vi "Start Calibrate.vi"(0 "CART TCP Connection In":refnum<k5>, 5 "Send Cal Command?":bool=TRUE, 7 "Calibrate Config":T1={"Frequency, MHz"=2412, "TX Gain"=0, "Data Rate"="1,0,0", "Packet Length"=4, "Packet Count"=4}, 11 "error in (no error)":errorcluster) -> (4 "CART TCP Connection Out":refnum<k5>, 6 "Messages Logged":string[](array[string]), 8 "More Pwr Reporting?":bool, 14 "Command Sent":string, 15 "error out":errorcluster)   [LabVIEW 2011]
uses:
  WLAN/UUT/QCA/Controls/QCA NART Response Type.ctl
  WLAN/UUT/QCA/NART Constants.vi
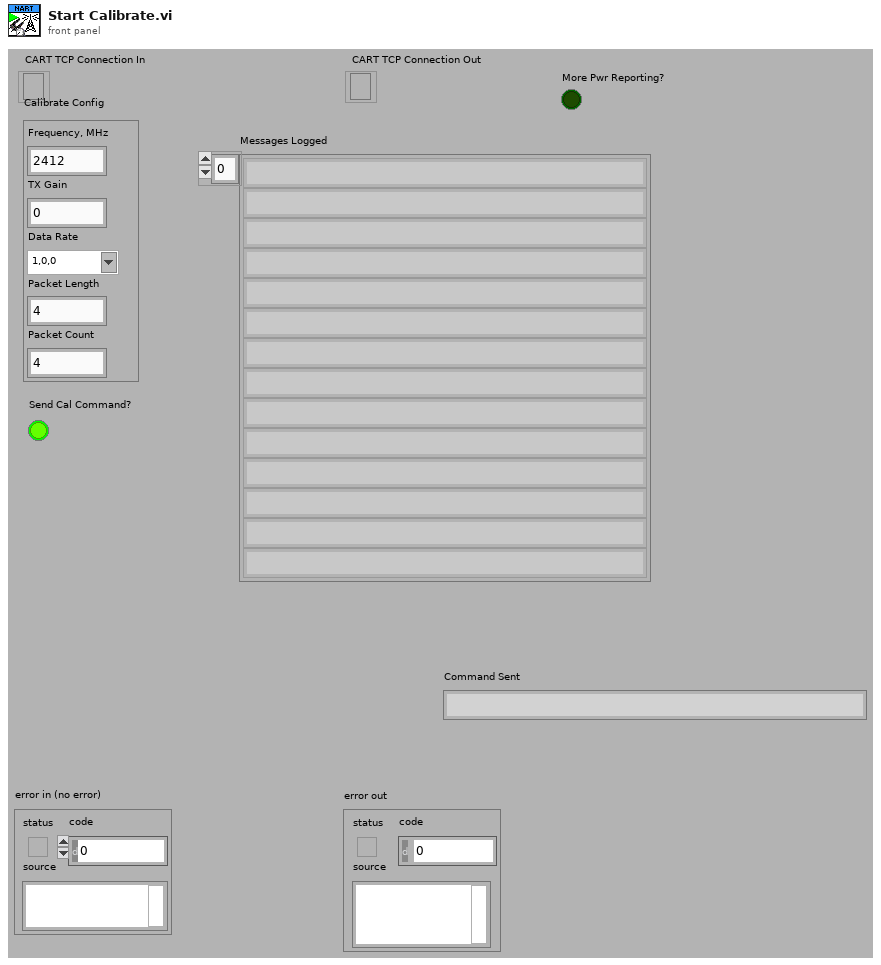
[diagram p1: front panel]
types:
  T1 = cluster{"Frequency, MHz":u32, "TX Gain":u32, "Data Rate":string, "Packet Length":u32, "Packet Count":i32}
  T2 = typedef "QCA NART Response Type.ctl" = enum16{"DEBUG", "CONTROL", "INFO", "WARNING", "ERROR", "NONE"}
  T3 = enum16{"none", "combined", "isolated", "iterate-combined ", "iterate-isolated"}
  T4 = cluster{"Name":string, "Type":enum16{"decimal", "string", "float", "hex"}}[]
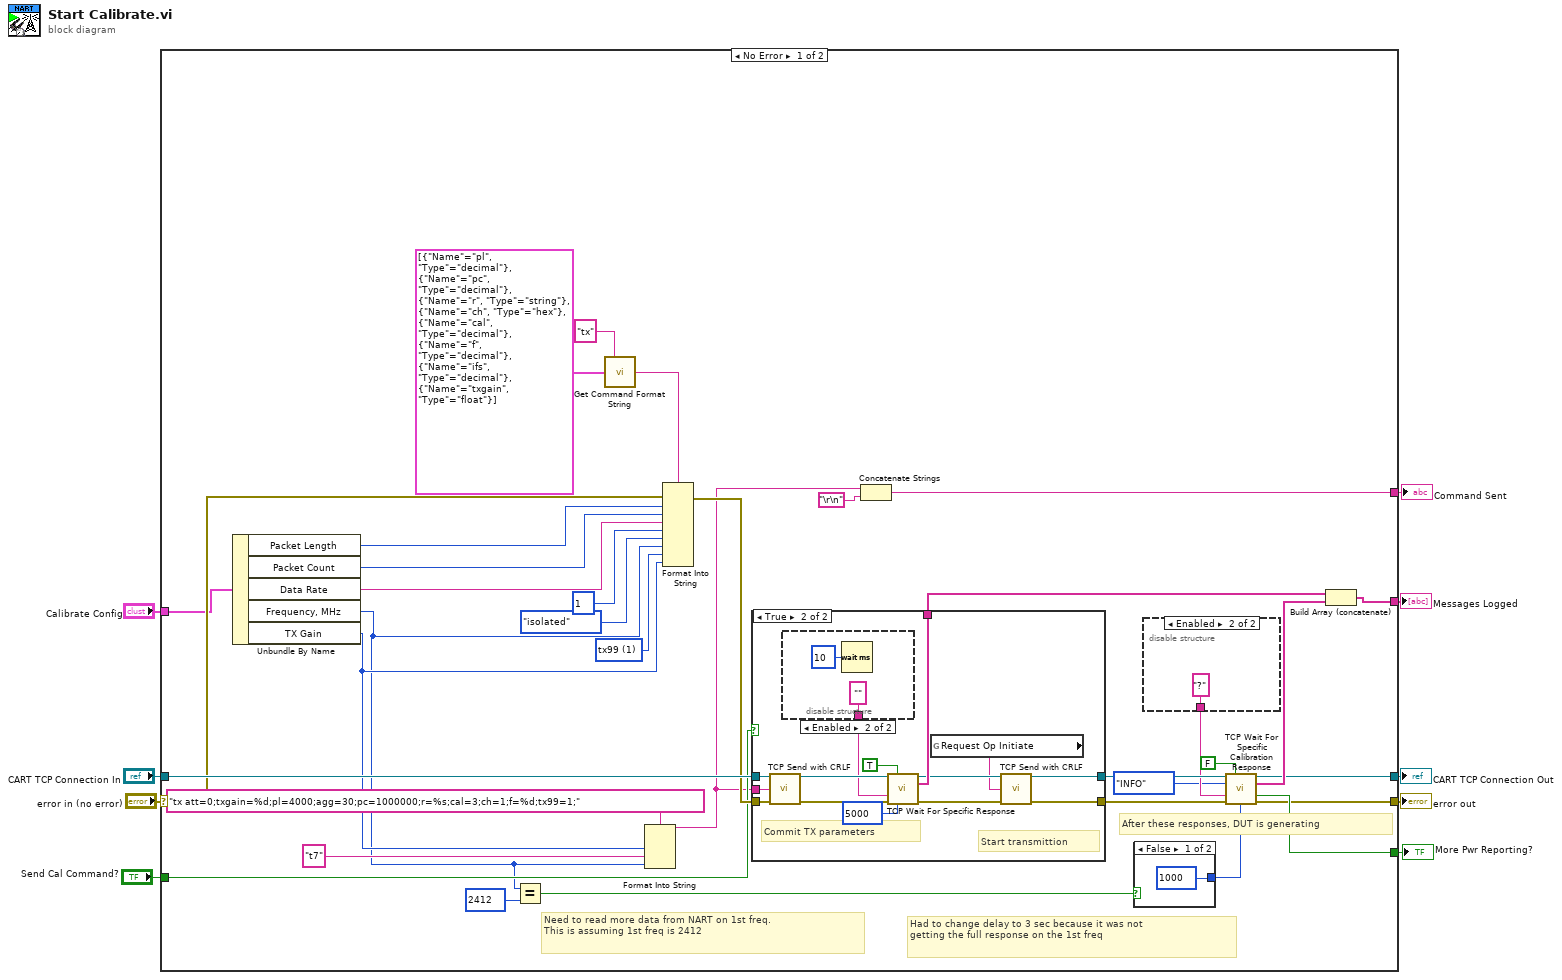
[diagram p0: block diagram]
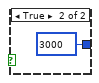
[diagram p2: hidden frame]
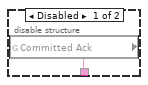
[diagram p4: hidden frame]
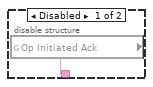
[diagram p5: hidden frame]
diagram:
  n1 = case shown="No Error" "error in (no error)" {
    selector: "error in (no error)" -> [w43 w69]
    tunnel: [w15 w69] -> w8
    tunnel: "CART TCP Connection In" -> [w44 w68]
    tunnel: [w16 w68] -> w6
    tunnel: "Calibrate Config" -> [w41 _]
    tunnel: [w37 _] -> w4
    tunnel: [w30 _] -> w3
    tunnel: [w18 _] -> w2
    tunnel: "Send Cal Command?" -> [w14 _]
    frame No Error {
      w28 = i16 1 items=["Regular"=-1, "tx100"=0, "tx99"=1] ("Inter Frame Spacing")
      # "Need to read more data from NART on 1st freq.\nThis is assuming 1st freq is 2412"
      # "Had to change delay to 3 sec because it was not \ngetting the full response on the 1st freq"
      # "After these responses, DUT is generating"
      n2 = Unbundle By Name(w41) -> ("Packet Length"=w40:u32, "Packet Count"=w34:i32, "Data Rate"=w21:string, "Frequency, MHz"=w12:u32, "TX Gain"=w22:u32)
      n3 = Equal?(x=w12, y=2412) -> (x = y?=w11:bool)
      n4 = call "Get Command Format String.vi"("Command"="tx", "Parameters"=T4 [{"Name"="pl", "Type"=enum."decimal"}, {"Name"="pc", "Type"=enum."decimal"}, {"Name"="r", "Type"=enum."string"}, {"Name"="ch", "Type"=enum."hex"}, {"Name"="cal", "Type"=enum."decimal"}, {"Name"="f", "Type"=enum."decimal"}, {"Name"="ifs", "Type"=enum."decimal"}, {"Name"="txgain", "Type"=enum."float"}]) -> ("Command Format String"=w31:string)  [unwired: 13 in]
      n5 = Format Into String(format string="tx att=0;txgain=%d;pl=4000;agg=30;pc=1000000;r=%s;cal=3;ch=1;f=%d;tx99=1;" ("Name"), w22, "t7" ("input 2"), w12) -> (resulting string=w10:string)  [unwired: 2 in, 1 out]
      n6 = Format Into String(format string=w31, error in=w43, w40, w34, w21, u32 1 ("Chains"), T3."isolated" ("Calibrate TXP"), w12, w28, w22) -> (error out=w42:errorcluster)  [unwired: 1 in, 1 out]
      n7 = case shown="True" w14 {
        tunnel: w44 -> [w47 w62]
        tunnel: w42 -> [w48 w61]
        tunnel: [_ w59] -> w39
        tunnel: [w47 w54] -> w36
        tunnel: [w48 w53] -> w35
        tunnel: w10 -> [_ w49]
        frame False {
        }
        frame True {
          # "Start transmittion"
          # "Commit TX parameters"
          n8 = call "TCP Send with CRLF.vi"("CART TCP Connection"=w62, "data in"=w49, "error IO"=w61) -> ("CART TCP Connection Out"=w58:refnum<k5>, "error out"=w57:errorcluster)  [unwired: 11 in]
          n9 = disable-structure shown="Enabled" {
            disable-tunnel: [w63 "" ("Expected Message Start (\"\":any)")] -> w50
            frame Disabled {
              n10 = global read "NART Constants.vi" "Committed Ack"() -> (w63:string)
            }
            frame Enabled {
              n11 = Wait (ms)(milliseconds to wait=u32 10) -> ()  [unwired: 1 out]
            }
          }
          n12 = call "TCP Wait For Specific Response.vi"("TCP Connection In"=w58, "Next response (t)"=TRUE, "Expected Message Start (\"\":any)"=w50, "error in"=w57, "Timeout (250 ms)"=5000 ("Timeout (100ms)")) -> ("TCP Connection Out"=w55:refnum<k5>, "TCP Messages"=w59:string[], "error out"=w56:errorcluster)  [unwired: 7 in, 1 out]
          n13 = global read "NART Constants.vi" "Request Op Initiate"() -> (w51:string)
          n14 = call "TCP Send with CRLF.vi"("CART TCP Connection"=w55, "data in"=w51, "error IO"=w56) -> ("CART TCP Connection Out"=w54:refnum<k5>, "error out"=w53:errorcluster)  [unwired: 11 in]
        }
      }
      n15 = Concatenate Strings(w10, "\r\n") -> (w30:string)
      n16 = case shown="False" w11 {
        tunnel: [1000 ("Timeout (250 ms)") 3000 ("Timeout (250 ms)")] -> w19
        frame False {
        }
        frame True {
        }
      }
      n17 = disable-structure shown="Enabled" {
        disable-tunnel: [w66 "?" ("Expected Message Start (\"\":any)")] -> w24
        frame Disabled {
          n18 = global read "NART Constants.vi" "Op Initiated Ack"() -> (w66:string)
        }
        frame Enabled {
        }
      }
      n19 = call "TCP Wait For Specific Calibration Response.vi"("TCP Connection In"=w36, "Next response (t)"=FALSE, "Expected Type"=QCA_NART_Response_Type."INFO", "Expected Message Start (\"\":any)"=w24, "error in"=w35, "Timeout (250 ms)"=w19) -> ("TCP Connection Out"=w16:refnum<k5>, "TCP Messages"=w38:string[], "More Pwr Reporting?"=w18:bool, "error out"=w15:errorcluster)  [unwired: 5 in, 1 out]
      n20 = Build Array (concatenate)(w39, w38) -> (w37:string[])
    }
    frame Error {
    }
  }
  "error out" <- w8
  "CART TCP Connection Out" <- w6
  "Messages Logged" <- w4
  "Command Sent" <- w3
  "More Pwr Reporting?" <- w2
